vi "Robot Global Data.vi"() -> ()   [LabVIEW 2012]
doc: "This global VI can contain as many global variables as you need. Place a control on the panel, give it a good name. To read or write to it from a VI, drag the icon to the diagram of that VI. You can also drag from the project. Click on the node to change which global you access. You shouldn't have multiple locations writing to a global or it will cause a race-condition."
uses:
  <vilib>/Rock Robotics/WPI/Camera/WPI_CameraImageSize.ctl
panel:
  out "Speed":dbl[](array[numeric])=[657.2927631578947, 0.0] format="%#_4f"
  out "New Robot":bool
  out "Loop Timer":dbl
  out "Inside Perimeter Catcher":bool
  out "Inside Perimeter Shooter":bool
  out "Rear Sonar OK":bool
  out "Front Sonar OK":bool
  out "Distance":dbl[](array[numeric])=[657.2927631578947, 0.0] format="%#_4f"
  in  "Reset Encoder":bool
  out "Gyro\nAngle":dbl
  in  "Reset Gyro\nZero Position":bool
  out "Target Info":T1(array[cluster])
  out "Pitch Calib. Factor":dbl=-6.0
  out "Feet/Second at FT":dbl=350.0
  in  "LED toggle rate (ms)":u32=100
  in  "image size":T2=enum."320x240"
  in  "Enable Vision":bool
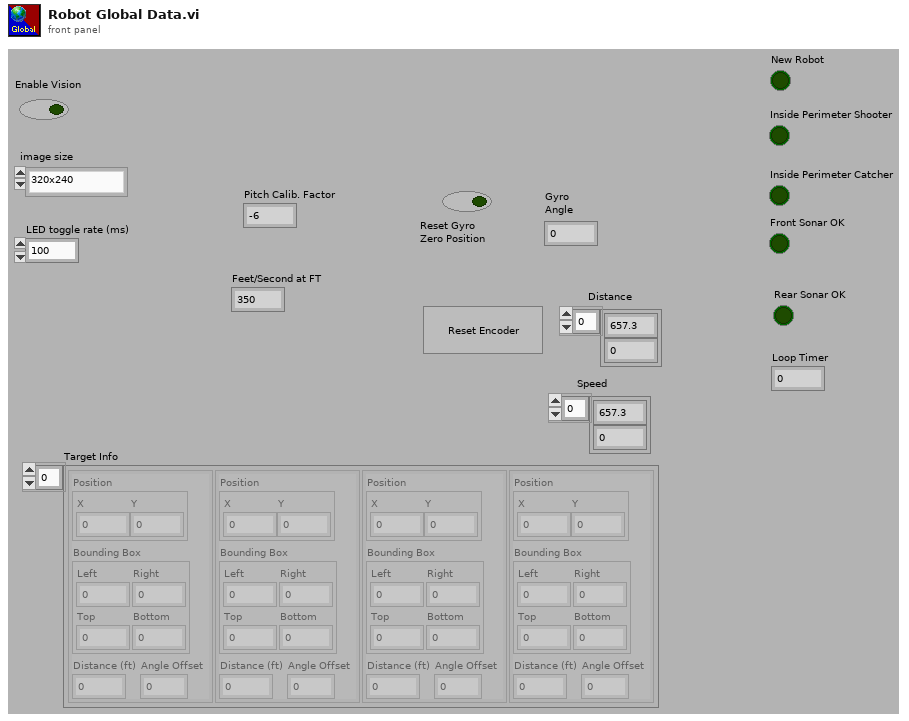
[diagram p1: front panel]
types:
  T1 = cluster{"Position":cluster{"X":dbl, "Y":dbl}, "Distance (ft)":dbl, "Angle Offset":dbl, "Bounding Box":cluster{"Left":dbl, "Top":dbl, "Right":dbl, "Bottom":dbl}}[]
  T2 = typedef "WPI_CameraImageSize.ctl" = enum16{"640x480", "320x240", "160x120"}
diagram:
